vi "Popup Menu.vi"(0 "Calling VI Ref":refnum<vi>, 5 "Initial Menu Options":string[](array[string]), 7 "Left":i16=600, 9 "Top":i16=300, 11 "String Ctrl Ref":refnum<vi>) -> (4 "Selection":string)   [LabVIEW 2020]
uses:
  <vilib>/Utility/miscctls.llb/LVPointTypeDef.ctl
  <vilib>/Utility/miscctls.llb/LVRectTypeDef.ctl
  <vilib>/event_ctls.llb/eventvkey.ctl
panel:
  in  "Tag 20":bool
  in  "Tag 19":bool
  in  "Tag 18":bool
  in  "Tag 17":bool
  in  "Tag 16":bool
  in  "Tag 15":bool
  in  "Tag 14":bool
  in  "Tag 13":bool
  in  "Tag 12":bool
  in  "Tag 11":bool
  in  "Tag 10":bool
  in  "Tag 9":bool
  in  "Tag 8":bool
  in  "Tag 7":bool
  in  "Tag 6":bool
  in  "Tag 5":bool
  in  "Tag 4":bool
  in  "Tag 3":bool
  in  "Tag 2":bool
  in  "Tag 1":bool
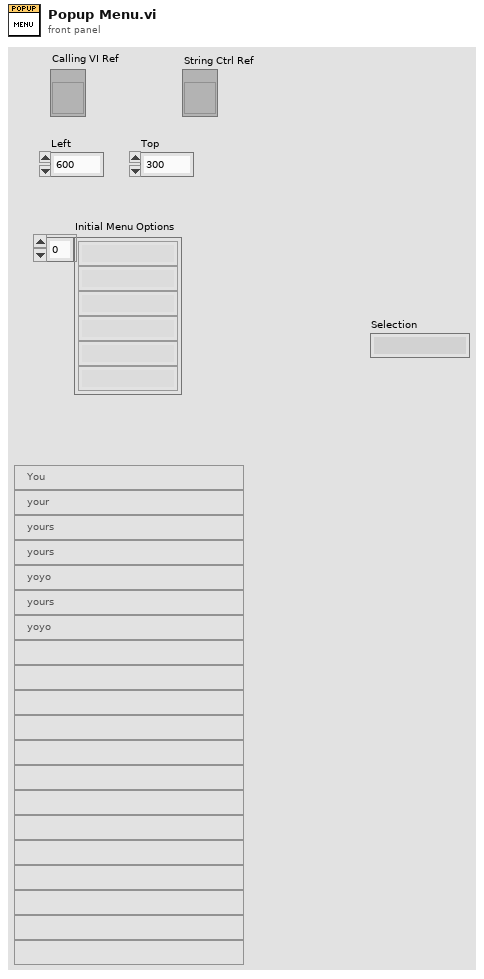
[diagram p1: front panel]
types:
  T1 = enum32{"Invalid", "Standard", "Closed", "Hidden", "Minimized", "Maximized"}
  T2 = typedef "LVRectTypeDef.ctl" = cluster{"Left":i16, "Top":i16, "Right":i16, "Bottom":i16}
  T3 = typedef "LVPointTypeDef.ctl" = cluster{"Horizontal":i16, "Vertical":i16}
  T4 = typedef "eventvkey.ctl" = enum16{"ASCII", "Enter", "Return", "Shift", "Ctrl", "Alt", "Cmd", "Opt", "Caps", "NumLock", "Clear", "Break", "Up", "Down", "Left", "Right", "Insert", "Delete", "Home", "End", "PageUp", "PageDown", "Escape", "Help", "Pause", "ScrollLock", "F1", "F2", "F3", "F4", "F5", "F6", "F7", "F8", "F9", "F10", "F11", "F12", "F13", "F14", "F15", "F16", "F17", "F18", "F19", "F20", "F21", "F22", "F23", "F24", "Play", "VolumeUp", "VolumeDown", "Mute", "Two Byte Char"}
  T5 = enum16{"Always On", "Always Off", "Off While Running"}
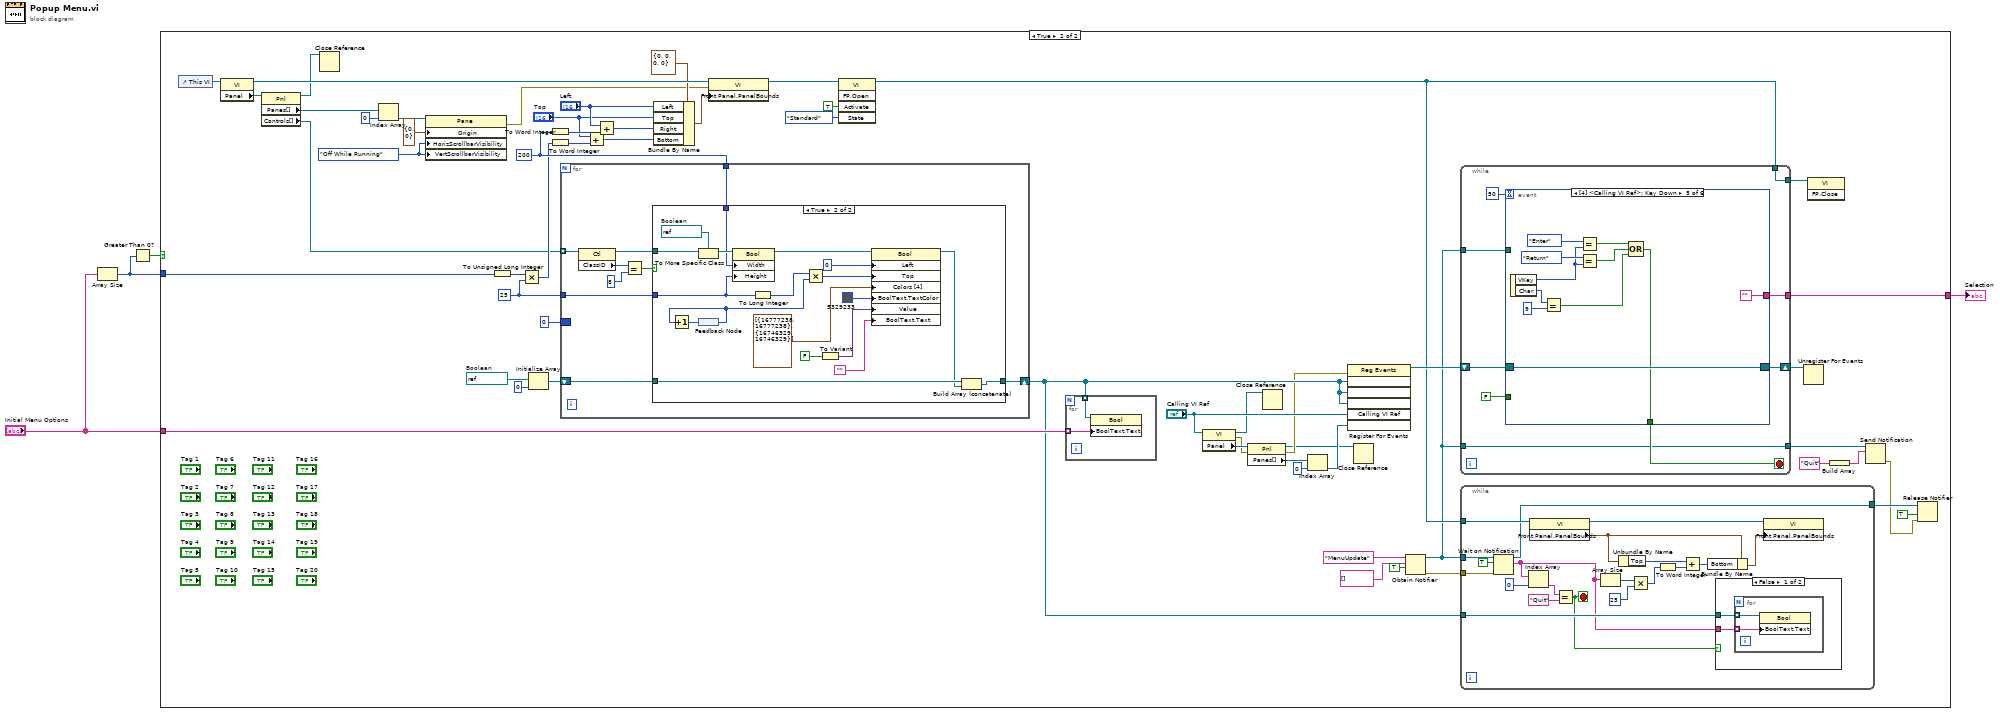
[diagram p0: block diagram]
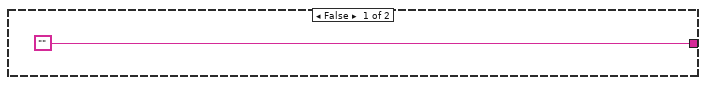
[diagram p2: hidden frame]
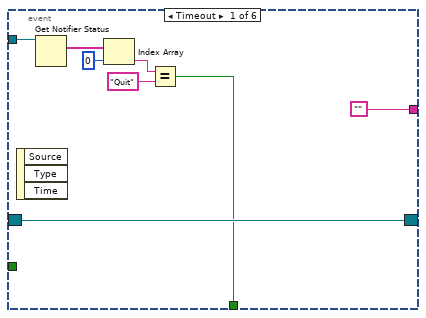
[diagram p4: hidden frame]
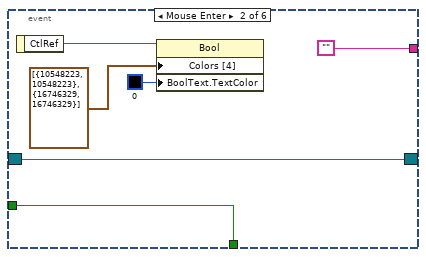
[diagram p5: hidden frame]
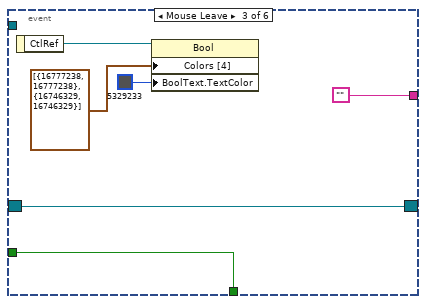
[diagram p6: hidden frame]
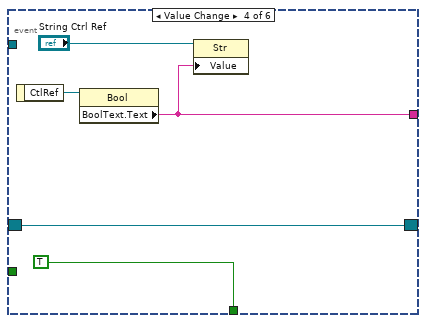
[diagram p7: hidden frame]
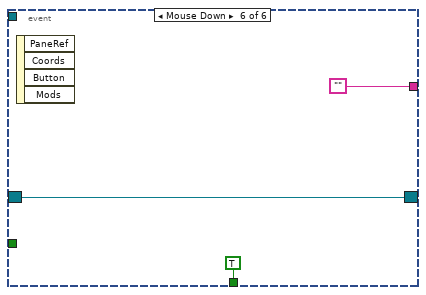
[diagram p8: hidden frame]
diagram:
  n1 = Array Size(array="Initial Menu Options") -> (size(s)=w2:i32)
  n2 = Greater Than 0?(x=w2) -> (x > 0?=w1:bool)
  n3 = case shown="True" w1 {
    tunnel: w2 -> [_ w34]
    tunnel: "Initial Menu Options" -> [_ w33]
    tunnel: ["" w31] -> w3
    frame False {
    }
    frame True {
      w46 = u32 25 ("Button Size:Height")
      w47 = u32 200 ("Button Size:Width")
      w57 = T5."Off While Running" ("Vertical Scrollbar Visibility")
      w61 = refnum<vi> refnum  # Boolean
      n4 = control-ref of="This VI"() -> (w51:refnum<vi>)
      n5 = property class="VI"(reference=w51) -> (reference out=w44:refnum<vi>, "Panel"=w52:refnum<vi>)  [unwired: 1 in, 1 out]
      n6 = property class="Pnl"(reference=w52) -> (reference out=w38:refnum<vi>, "Panes[]"=w55:refnum<vi>[], "Controls[]"=w39:refnum<vi>[])  [unwired: 1 in, 1 out]
      n7 = Close Reference(reference=w38) -> ()  [unwired: 1 in, 1 out]
      n8 = Index Array(array=w55, index=0) -> (element=w54:refnum<vi>)
      n9 = property class="Pane"(reference=w54, "Origin"=T3 {"Horizontal"=0, "Vertical"=0}, "HorizScrollbarVisibility"=w57, "VertScrollbarVisibility"=w57) -> (error out=w13:errorcluster)  [unwired: 1 in, 1 out]
      n10 = To Unsigned Long Integer(number=w34) -> (unsigned 32bit integer=w32:u32)
      n11 = Multiply(x=w32, y=w46) -> (x*y=w45:u32)
      n12 = Initialize Array(w61, 0 ("dimension size")) -> (w59:refnum<vi>[])
      n13 = To Word Integer(number=w47) -> (16bit integer=w58:i16)
      n14 = To Word Integer(number=w45) -> (16bit integer=w50:i16)
      n15 = for {
        tunnel: w39 -> [w146] mode=indexing
        shift-right: [w140] -> w20
        shift-left: w59 -> [w141]
        tunnel: w47 -> [w139]
        tunnel: w46 -> [w138]
        border: 0 ("Button Size:Height") -> [_]
        n16 = property class="Ctl"(reference=w146) -> (reference out=w142:refnum<vi>, "ClassID"=w145:u32)  [unwired: 1 in, 1 out]
        n17 = Equal?(x=w145, y=u32 8) -> (x = y?=w143:bool)
        n18 = case shown="True" w143 {
          tunnel: w142 -> [_ w159]
          tunnel: w141 -> [w147 w158]
          tunnel: [w147 w156] -> w140
          tunnel: w139 -> [_ w153]
          tunnel: w138 -> [_ w152]
          frame False {
          }
          frame True {
            w166 = refnum<vi> refnum  # Boolean
            n19 = To More Specific Class(target class=w166, reference=w159) -> (specific class reference=w155:refnum<vi>)  [unwired: 1 in, 1 out]
            n20 = feedback #1() -> (w148:i32)
            n21 = Increment(x=w148) -> (x+1=w149:i32)
            n22 = feedback-in #1(w149) -> ()
            n23 = property class="Bool"(reference=w155, "Width"=w153, "Height"=w152) -> (reference out=w154:refnum<vi>)  [unwired: 1 in, 1 out]
            n24 = To Long Integer(number=w152) -> (32bit integer=w151:i32)
            n25 = Multiply(x=w151, y=w148) -> (x*y=w164:i32)
            n26 = To Variant(anything=FALSE) -> (Variant=w160:variant)
            n27 = property class="Bool"(reference=w154, "Left"=0 ("Position:Left"), "Top"=w164, "Colors [4]"=cluster{u32, u32}[] [{16777238, 16777238}, {16746329, 16746329}], "BoolText.TextColor"=u32 5329233 ("Boolean Text.Colors:FG Color"), "Value"=w160, "BoolText.Text"="") -> (reference out=w157:refnum<vi>)  [unwired: 1 in, 1 out]
            n28 = Build Array (concatenate)(w158, w157) -> (w156:refnum<vi>[])
          }
        }
      }
      n29 = Add(x="Top", y=w50) -> (x+y=w48:i16)
      n30 = Add(x="Left", y=w58) -> (x+y=w49:i16)
      n31 = Bundle By Name(cluster=T2 {"Left"=0, "Top"=0, "Right"=0, "Bottom"=0} ("Front Panel Window:Panel Bounds"), "Left"="Left", "Top"="Top", "Right"=w49, "Bottom"=w48) -> (w40:T2)
      n32 = property class="VI"(reference=w44, error in=w13, "Front Panel.PanelBounds"=w40) -> (reference out=w37:refnum<vi>)  [unwired: 1 out]
      n33 = invoke class="VI" method="FP.Open"(reference=w37, "Activate"=TRUE ("Activate?"), "State"=T1."Standard") -> (reference out=w22:refnum<vi>)  [unwired: 2 in, 4 out]
      n34 = for {
        tunnel: w33 -> [w88] mode=indexing
        tunnel: w20 -> [w89] mode=indexing
        n35 = property class="Bool"(reference=w89, "BoolText.Text"=w88) -> ()  [unwired: 1 in, 2 out]
      }
      n36 = property class="VI"(reference="Calling VI Ref") -> (reference out=w8:refnum<vi>, error out=w12:errorcluster, "Panel"=w28:refnum<vi>)  [unwired: 1 in]
      n37 = property class="Pnl"(reference=w28, error in=w12) -> (reference out=w9:refnum<vi>, error out=w11:errorcluster, "Panes[]"=w27:refnum<vi>[])
      n38 = Close Reference(reference=w8) -> ()  [unwired: 1 in, 1 out]
      n39 = Index Array(array=w27, index=0) -> (element=w10:refnum<vi>)
      n40 = register-events(error in=w11, w20, w20, w20, "Calling VI Ref", w10) -> (reference out=w63:refnum<event-registration>)  [unwired: 1 in, 1 out]
      n41 = Close Reference(reference=w9) -> ()  [unwired: 1 in, 1 out]
      n42 = Obtain Notifier(name (unnamed)="MenuUpdate", notification data type=string[] [], create if not found? (T)=TRUE) -> (notifier out=w7:refnum<notifier>, error out=w21:errorcluster)  [unwired: 1 in, 1 out]
      n43 = while {
        shift-right: [w97] -> w62
        shift-left: w63 -> [w98]
        tunnel: [w94] -> w31
        tunnel: w22 -> [w93]
        tunnel: [w93] -> w30
        tunnel: w7 -> [w92]
        tunnel: [w92] -> w17
        tunnel: w7 -> [w90]
        stop <- w96 stop-if-true
        n44 = event shown="[4] <Calling VI Ref>: Key Down" {
          selector: w98 -> [w106 w110 w113 w123 w130 w137]
          dyn-events: [w106 w110 w113 w123 w130 w137] -> w97
          timeout: 50 -> [_ _ _ _ _ _]
          tunnel: [w99 w109 w116 TRUE w126 TRUE] -> w96
          tunnel: FALSE -> [_ w109 w116 _ _ _]
          tunnel: ["" "" "" w119 "" ""] -> w94
          tunnel: w90 -> [w104 _ _ _ _ _]
          event Timeout {
            n45 = event-data() -> ()  [unwired: 1 in, 3 out]
            n46 = Get Notifier Status(notifier=w104) -> (current notification=w103:string[])  [unwired: 1 in, 4 out]
            n47 = Index Array(array=w103, index=0) -> (element=w100:string)
            n48 = Equal?(x=w100, y="Quit") -> (x = y?=w99:bool)
          }
          event Mouse Enter {
            n49 = event-data() -> ("CtlRef"=w111:refnum<vi>)  [unwired: 1 in]
            n50 = property class="Bool"(reference=w111, "Colors [4]"=cluster{u32, u32}[] [{10548223, 10548223}, {16746329, 16746329}], "BoolText.TextColor"=u32 0 ("Boolean Text.Colors:FG Color")) -> ()  [unwired: 1 in, 2 out]
          }
          event Mouse Leave {
            n51 = event-data() -> ("CtlRef"=w117:refnum<vi>)  [unwired: 1 in]
            n52 = property class="Bool"(reference=w117, "Colors [4]"=cluster{u32, u32}[] [{16777238, 16777238}, {16746329, 16746329}], "BoolText.TextColor"=u32 5329233 ("Boolean Text.Colors:FG Color")) -> ()  [unwired: 1 in, 2 out]
          }
          event Value Change {
            n53 = event-data() -> ("CtlRef"=w121:refnum<vi>)  [unwired: 1 in]
            n54 = property class="Bool"(reference=w121) -> ("BoolText.Text"=w119:string)  [unwired: 1 in, 2 out]
            n55 = property class="Str"(reference="String Ctrl Ref", "Value"=w119) -> ()  [unwired: 1 in, 2 out]
          }
          event Key Down {
            n56 = event-data() -> ("VKey"=w131:T4, "Char"=w129:i16)  [unwired: 1 in]
            n57 = Equal?(x=w129, y=i16 9) -> (x = y?=w125:bool)
            n58 = Equal?(x=eventvkey."Enter" ("VKey"), y=w131) -> (x = y?=w127:bool)
            n59 = Equal?(x=eventvkey."Return" ("VKey"), y=w131) -> (x = y?=w124:bool)
            n60 = Compound Arithmetic op=OR(w127, w124, w125) -> (w126:bool)
          }
          event Mouse Down {
            n61 = event-data() -> ()  [unwired: 1 in, 4 out]
          }
        }
      }
      n62 = while {
        tunnel: w22 -> [w71]
        tunnel: w7 -> [w83]
        tunnel: w21 -> [w82]
        tunnel: w20 -> [w68]
        tunnel: [w66] -> w19
        stop <- w64 stop-if-true
        n63 = Wait on Notification(notifier=w83, ignore previous (F)=TRUE, error in (no error)=w82) -> (notifier out=w66:refnum<notifier>, notification=w67:string[])  [unwired: 1 in, 2 out]
        n64 = Index Array(array=w67, index=0) -> (element=w80:string)
        n65 = property class="VI"(reference=w71) -> (reference out=w73:refnum<vi>, "Front Panel.PanelBounds"=w74:T2)  [unwired: 1 in, 1 out]
        n66 = Equal?(x=w80, y="Quit") -> (x = y?=w64:bool)
        n67 = Array Size(array=w67) -> (size(s)=w78:i32)
        n68 = Unbundle By Name(w74) -> ("Top"=w75:i16)
        n69 = Multiply(x=w78, y=25) -> (x*y=w70:i32)
        n70 = To Word Integer(number=w70) -> (16bit integer=w69:i16)
        n71 = Add(x=w75, y=w69) -> (x+y=w76:i16)
        n72 = Bundle By Name(cluster=w74, "Bottom"=w76) -> (w72:T2)
        n73 = case shown="False" w64 {
          tunnel: w68 -> [w85 _]
          tunnel: w67 -> [w84 _]
          frame False {
            n74 = for {
              tunnel: w84 -> [w87] mode=indexing
              tunnel: w85 -> [w86] mode=indexing
              n75 = property class="Bool"(reference=w86, "BoolText.Text"=w87) -> ()  [unwired: 1 in, 2 out]
            }
          }
          frame True {
          }
        }
        n76 = property class="VI"(reference=w73, "Front Panel.PanelBounds"=w72) -> ()  [unwired: 1 in, 2 out]
      }
      n77 = Unregister For Events(event registration refnum=w62) -> ()  [unwired: 1 in, 1 out]
      n78 = invoke class="VI" method="FP.Close"(reference=w30) -> ()  [unwired: 2 in, 3 out]
      n79 = Build Array("Quit") -> (w15:string[])
      n80 = Send Notification(notification=w15, notifier=w17) -> (error out=w6:errorcluster)  [unwired: 1 in, 1 out]
      n81 = Release Notifier(notifier=w19, force destroy? (F)=TRUE, error in (no error)=w6) -> ()  [unwired: 3 out]
    }
  }
  "Selection" <- w3
